vi "VCS Set Gateway Settings.vi"(8 "error in (no error)":errorcluster, 10 "Baudrate":u32, 11 "keyHandle in":u32) -> (0 "error out":errorcluster, 3 "keyHandle out":u32)   [LabVIEW 2018]
doc: "<B>VCS Set Gateway Settings</B> writes the gateway communication parameters. For correct communication, use the same baud rate as the connected device."
uses:
  Resources/EposCmd64.dll
  Resources/EposCmd.dll
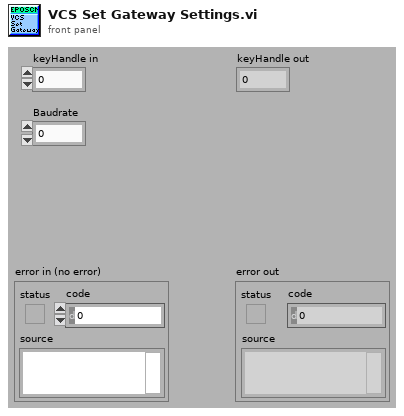
[diagram p1: front panel]
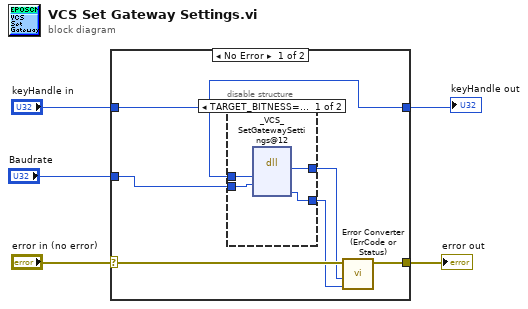
[diagram p0: block diagram]
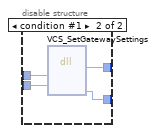
[diagram p2: hidden frame]
diagram:
  n1 = case shown="No Error" "error in (no error)" {
    selector: "error in (no error)" -> [w11 w21]
    tunnel: [w10 w21] -> w4
    tunnel: "keyHandle in" -> [w8 w20]
    tunnel: [w8 w20] -> w2
    tunnel: "Baudrate" -> [w6 _]
    frame No Error {
      n2 = disable-structure shown="TARGET_BITNESS==32, Standard" {
        disable-tunnel: [w15 w19] -> w9
        disable-tunnel: w8 -> [w14 w18]
        disable-tunnel: [w13 w17] -> w7
        disable-tunnel: w6 -> [w12 w16]
        frame condition #0 (active) {
          n3 = dll-call lib="C:/Projeto em LabVIEW/EPOS-LabVIEW-Instrument-Driver-En/LabVIEW/maxon EPOS/Resources/EposCmd.*" fn="_VCS_SetGatewaySettings@12" ("EposCmd.dll:_VCS_SetProtocolStackSettings@16")("KeyHandle"=w14, "Baudrate"=w12) -> ("Rückgabetyp"=w13:i32, "pErrorCode"=w15:u32)  [unwired: 6 in, 2 out]
        }
        frame condition #1 {
          n4 = dll-call lib="C:/Sources/LabView/maxon EPOS/Resources/EposCmd64.dll" fn="VCS_SetGatewaySettings" ("EposCmd.dll:_VCS_SetProtocolStackSettings@16")("KeyHandle"=w18, "Baudrate"=w16) -> ("return type"=w17:i32, "pErrorCode"=w19:u32)  [unwired: 6 in, 2 out]
        }
      }
      n5 = call "Error Converter (ErrCode or Status).vi"("error code"=w9, "return type"=w7, "error in (no error)"=w11) -> ("error out"=w10:errorcluster)  [unwired: 7 in]
    }
    frame Error {
    }
  }
  "error out" <- w4
  "keyHandle out" <- w2
